vi "get_binary_file.vi"(8 "error in":errorcluster, 11 "Sensor configuration":path) -> (0 "error out":errorcluster, 1 "Type":string, 2 "Channels":string, 3 "Binary File ref":refnum<file>, 5 "Stream dimensions":cluster{"x dimension":i32, "y dimension":i32})   [LabVIEW 2019, in "Lib_Simx.lvlib"]
doc: "Obtain the reference to the binary file to read based on the name of the sensor type and the custom name assigned by the user."
uses:
  Lib_Simx.lvlib
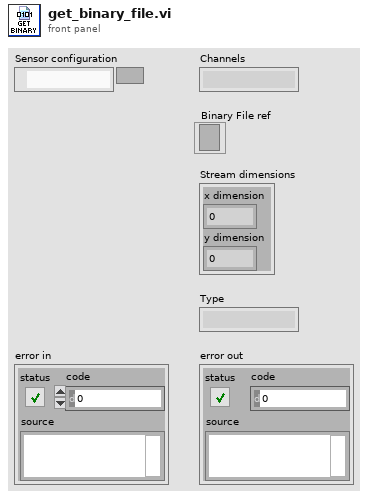
[diagram p1: front panel]
types:
  T1 = enum16{"open", "replace", "create", "open or create", "replace or create", "replace or create with confirmation"}
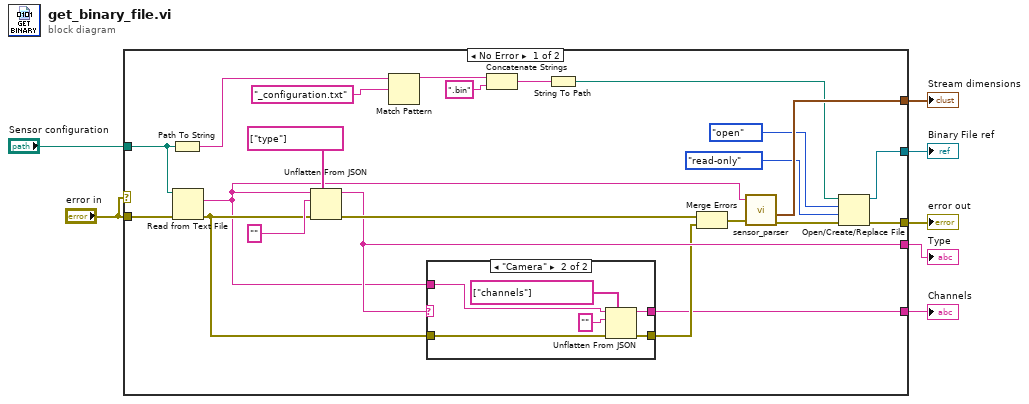
[diagram p0: block diagram]
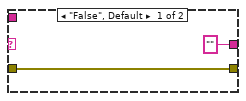
[diagram p2: hidden frame]
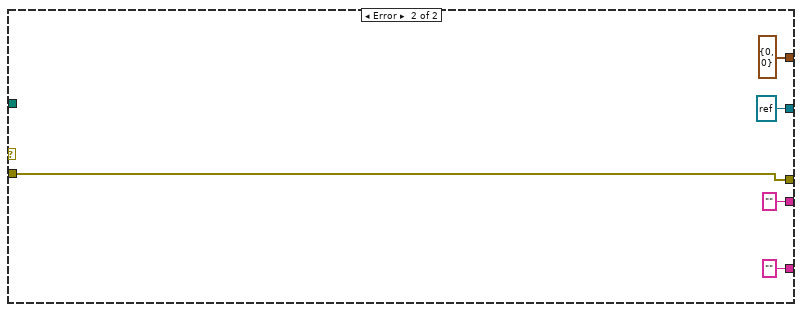
[diagram p3: hidden frame]
diagram:
  n1 = case shown="No Error" "error in" {
    tunnel: "error in" -> [w30 w41]
    tunnel: "Sensor configuration" -> [w29 _]
    tunnel: [w28 cluster{"x dimension":i32, "y dimension":i32} {"x dimension"=0, "y dimension"=0} ("Stream dimensions")] -> w6
    tunnel: [w15 w41] -> w5
    tunnel: [w13 ""] -> w3
    tunnel: [w9 ""] -> w2
    tunnel: [w8 refnum<file> refnum ("refnum out")] -> w1
    frame No Error {
      n2 = Path To String(path=w29) -> (string=w21:string)
      n3 = Read from Text File(file (use dialog)=w29, error in=w30) -> (text=w12:string, error out=w14:errorcluster)  [unwired: 2 in, 2 out]
      n4 = Unflatten From JSON(path=string[] ["type"], JSON string=w12, type and defaults="", error in (no error)=w14) -> (value=w13:string, error out=w26:errorcluster)  [unwired: 3 in]
      n5 = Match Pattern(string=w21, regular expression="_configuration.txt" ("string")) -> (before substring=w18:string)  [unwired: 1 in, 3 out]
      n6 = case shown="\"Camera\"" w13 {
        tunnel: w14 -> [w32 w38]
        tunnel: [w32 w37] -> w10
        tunnel: w12 -> [_ w36]
        tunnel: ["" w33] -> w9
        frame "False", Default {
        }
        frame "Camera" {
          n7 = Unflatten From JSON(path=string[] ["channels"], JSON string=w36, type and defaults="", error in (no error)=w38) -> (value=w33:string, error out=w37:errorcluster)  [unwired: 3 in]
        }
      }
      n8 = Concatenate Strings(w18, ".bin" ("string")) -> (w22:string)
      n9 = String To Path(string=w22) -> (path=w25:path)
      n10 = Merge Errors(w26, w10) -> (w11:errorcluster)
      n11 = call "sensor_parser.vi"("Sensor configuration"=w12, "error in"=w11) -> ("Stream dimensions"=w28:cluster{"x dimension":i32, "y dimension":i32}, "error out"=w27:errorcluster)  [unwired: 1 in, 2 out]
      n12 = Open/Create/Replace File(file path (use dialog)=w25, error in=w27, operation (0:open)=T1."open", access (0:read/write)=enum16{"read/write", "read-only", "write-only"}."read-only") -> (refnum out=w8:refnum<file>, error out=w15:errorcluster)  [unwired: 2 in, 1 out]
    }
    frame Error {
    }
  }
  "Stream dimensions" <- w6
  "error out" <- w5
  "Channels" <- w2
  "Type" <- w3
  "Binary File ref" <- w1
